vi "LV to ITX XY2 AutoPlot.vi"(0 "filename":string="filename", 1 "path":path=path "C:/", 5 "Notes":string, 7 "Data":cluster{"Y  Array":dbl[]}[](array[cluster]), 11 "wavenames (.Vx, etc)":string[](array[string])=["time", "x", "y", "z"], 12 "X,Y Labels":string[](array[string])=["x label", "y label"], 13 "X,Y Log":i32[](array[numeric]), 14 "input command string":string="Display/R '#wave#'\nAppendToGraph '#wave#'\nLabel bottom \"#labelX#\"\nLabel left \"#labelY#\"\nModifyGraph rgb('#wave#')=(#r#,#g#,#b#)\n\\\\s('#wave#') #label#\nModifyGraph mirror(bottom)=1\nModifyGraph width=216\nModifyGraph height={Aspect,0.6}\nModifyGraph Log(bottom)=#bottomlog#\nModifyGraph Log(left)=#leftlog#", 15 "error in":errorcluster) -> (4 "file":path, 10 "error out":errorcluster)   [LabVIEW 2016, in "LV to ITX.lvclass"]
doc: "Write data to ITX file. This AutoPlot VI adds commands to automatically create a graph in Igor to quickly view your data.\n\n-- path: base path to save data\n-- filename: base filename\n-- Notes: add any notes here to help you remember what experiment you did\n-- Data: Cluster array\n It is recommended that you make the first cluster an array of timestamps\n-- wavenames: Give each data array a unique name such as \"time, bias, current,...\"zz\n-- X,Y Labels: For plotting in Igor. Can be ignored.\n-- X,Y Log: Do you wan to show X or Y on Log scale in Igor?"
uses:
  LV to ITX.lvclass
  Typedefs/Filetype--enum.ctl
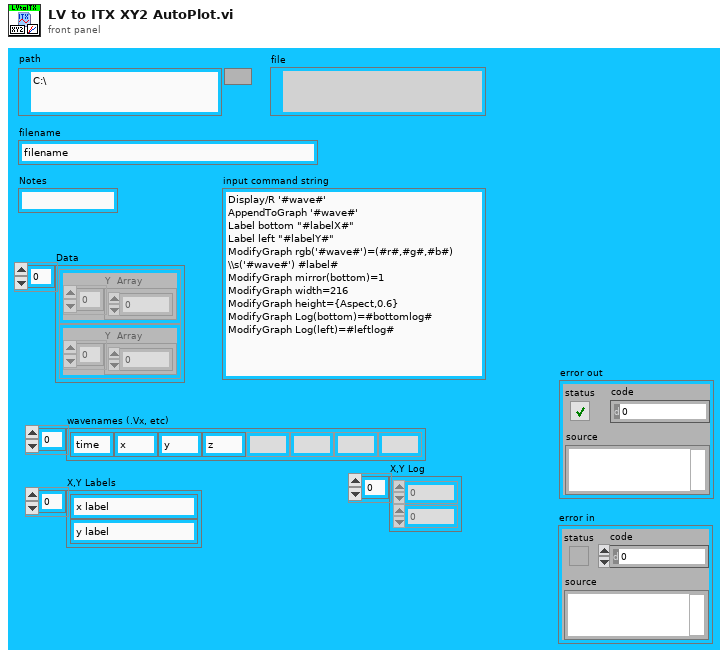
[diagram p1: front panel]
types:
  T1 = typedef "LV to ITX.lvclass/Filetype--enum.ctl" = enum16{"DAT", "ITX", "HDF5", "TDMS", "VI"}
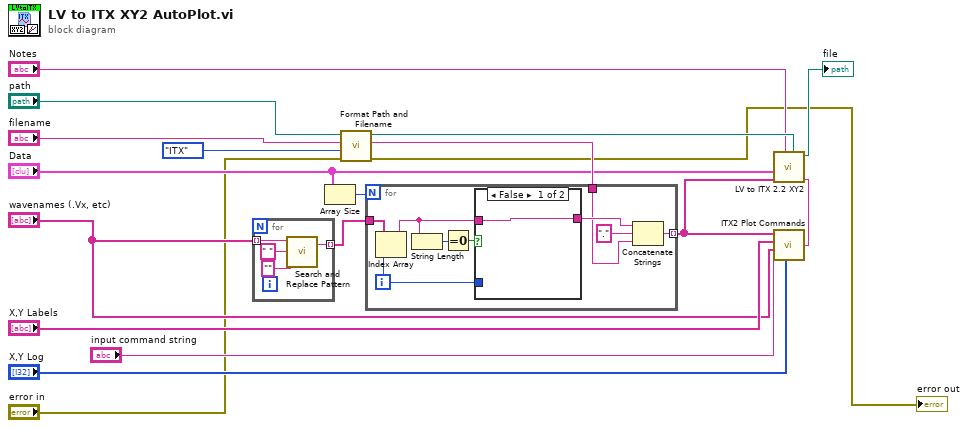
[diagram p0: block diagram]
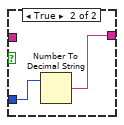
[diagram p2: hidden frame]
diagram:
  n1 = for {
    tunnel: "wavenames (.Vx, etc)" -> [w20] mode=indexing
    tunnel: [w19] -> w7 mode=indexing
    n2 = call <vilib>:"Search and Replace Pattern.vi"("string"=w20, "regular expression (\"\")"=" " ("regular expression (\"\")"), "replace string (\"\")"="" ("replace string (\"\")")) -> ("result string"=w19:string)  [unwired: 2 in, 1 out]
  }
  n3 = Array Size(array="Data") -> (size(s)=w17:i32)
  n4 = call "Format Path and Filename.vi"("error in"="error in", "Type (TDMS)"=Filetype--enum."ITX", "filename"="filename", "path"="path") -> ("error out"=→"error out":errorcluster, "filename without extension"=w16:string, "path"=w14:path)  [unwired: 5 in]
  n5 = for {
    N: w17 -> [_]
    tunnel: w7 -> [w26]
    tunnel: w16 -> [w23]
    tunnel: [w31] -> w5 mode=indexing
    i -> [w27]
    n6 = Index Array(array=w26, index=w27) -> (element=w25:string)
    n7 = String Length(string=w25) -> (length=w28:i32)
    n8 = Equal To 0?(x=w28) -> (x = 0?=w29:bool)
    n9 = case shown="False" w29 {
      tunnel: w27 -> [_ w33]
      tunnel: [w32 w34] -> w24
      tunnel: w25 -> [w32 _]
      frame False {
      }
      frame True {
        n10 = Number To Decimal String(number=w33) -> (decimal integer string=w34:string)  [unwired: 1 out]
      }
    }
    n11 = Concatenate Strings(w24, "." ("string"), w23) -> (w31:string)
  }
  n12 = call "ITX2 Plot Commands.vi"("X,Y Log"="X,Y Log", "input string"="input command string", "Plot labels"="wavenames (.Vx, etc)", "X,Y Labels"="X,Y Labels", "wavenames"=w5) -> ("result string"=w6:string)  [unwired: 1 in]
  n13 = call "LV to ITX 2.2 XY2.vi"("Commands"=w6, "filename"=w14, "Notes"="Notes", "wavenames"=w5, "array of clusters"="Data") -> ("file"=→"file":path)  [unwired: 6 in]
